vi "Update Method Result.vi"(8 "error in (no error)":errorcluster, 10 "Test Method Result":T1, 11 "Test Tree In":refnum<class "Test Result Tree V2.lvclass">) -> (0 "error out":errorcluster, 3 "Test Tree Out":refnum<class "Test Result Tree V2.lvclass">)   [LabVIEW 2020, in "Test Result Tree V2.lvclass"]
uses:
  Test Result Tree/Test Result Tree V2.lvclass
  C:/Git/astemes-lunit/source/Framework/Helper Classes/Test Tree/Test Tree.lvclass
  Framework/Result Types/Method Result/Method Result.ctl
  Result/Status.ctl
  Framework/Result Types/Assertion Result/Assertion Result.ctl
  Framework/Result Types/Assertion Result/Public/TypeDefs/Assertion Type.ctl
  Framework/Helper Classes/Test Tree/Test Tree.lvclass/Test Tree.ctl
  Test Result Tree/Test Result Tree V2.lvclass/Test Result Tree V2.ctl
  Framework/Result Types/Method Result/Method Result.lvlib
  Framework/Helper Classes/Test Tree/Test Tree.lvclass
  C:/Git/astemes-lunit/source/Rewrite Project/Test Result Tree/Test Result Tree/Test Result Tree V2.lvclass
  Framework/Result Types/Assertion Result/Assertion Result.lvlib
  Result/Result.lvlib
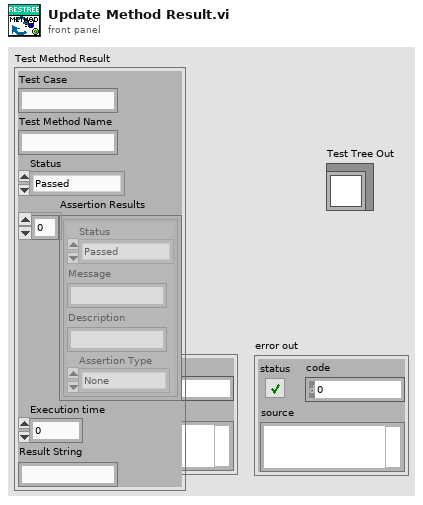
[diagram p1: front panel]
types:
  T1 = typedef "Method Result.lvlib/Method Result.ctl" = cluster{"Test Case":string, "Test Method Name":string, "Status":T2, "Assertion Results":T3[], "Execution time":dbl, "Result String":string}
  T2 = typedef "Result.lvlib/Status.ctl" = enum16{"Passed", "Failed", "Error", "Skipped", "Setup Error", "Broken", "Teardown Error"}
  T3 = typedef "Assertion Result.lvlib/Assertion Result.ctl" = cluster{"Status":T2, "Message":string, "Description":string, "Assertion Type":T4}
  T4 = typedef "Result.lvlib/Assertion Type.ctl" = enum16{"None", "Pass", "Fail", "Skip", "Pass if Equal", "Fail if Equal", "Pass if Error", "Fail if Error", "Pass if", "Fail if"}
  T5 = typedef "Assertion Result.lvlib/Status.ctl" = enum16{"Pass", "Fail", "Error", "Skipped", "Setup Error", "Broken", "Teardown Error"}
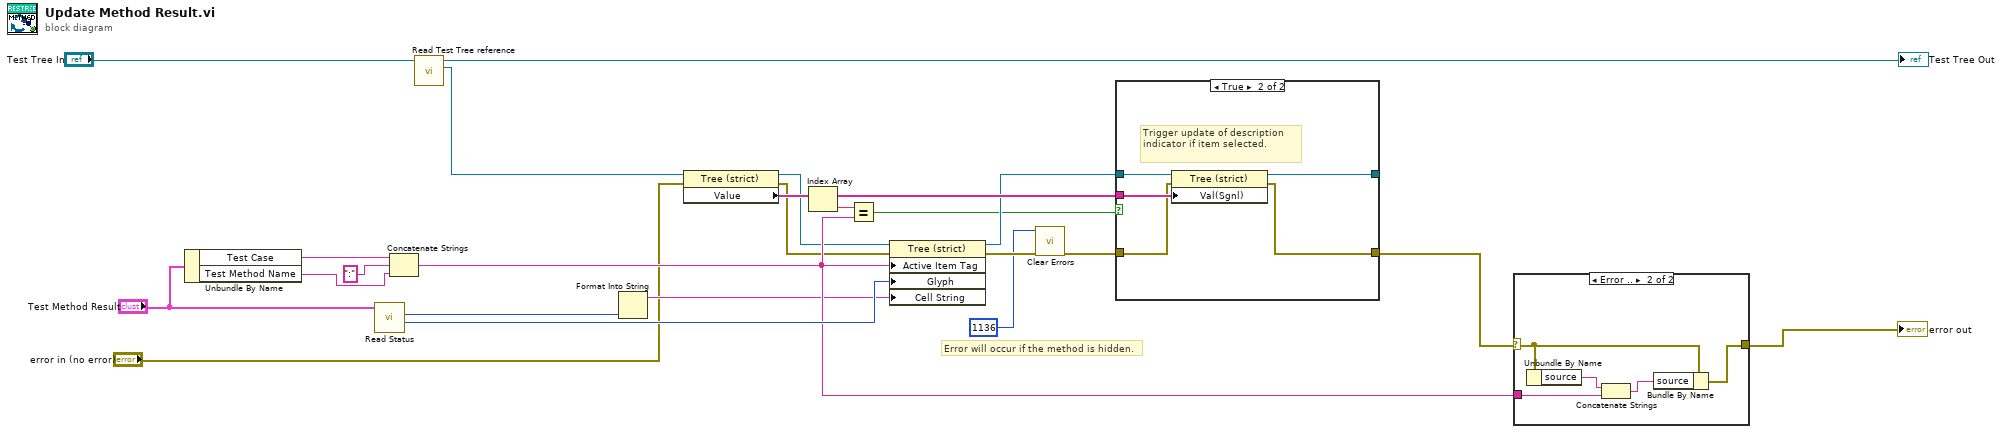
[diagram p0: block diagram]
diagram:
  # "Error will occur if the method is hidden."
  n1 = Unbundle By Name("Test Method Result") -> ("Test Case"=w1:string, "Test Method Name"=w2:string)
  n2 = call "Read Status.vi"("Method Result In"="Test Method Result") -> ("Glyph Index"=w21:i32, "Status"=w22:T5)  [unwired: 8 in, 1 out]
  n3 = Concatenate Strings(w1, ":" ("string"), w2) -> (w19:string)
  n4 = call "Read Test Tree reference.vi"("Test Tree in"="Test Tree In") -> ("Test Tree reference"=w5:refnum<vi>, "Test Tree out"=→"Test Tree Out":refnum<class "Test Result Tree V2.lvclass">)  [unwired: 8 in, 1 out]
  n5 = Format Into String(w22) -> (resulting string=w18:string)  [unwired: 3 in, 1 out]
  n6 = property on="Property Node" class="Tree (strict)"(reference=w5, error in="error in (no error)") -> (reference out=w11:refnum<vi>, error out=w12:errorcluster, "Value"=w16:string[])
  n7 = Index Array(array=w16) -> (element=w17:string)  [unwired: 1 in]
  n8 = Equal?(x=w17, y=w19) -> (x = y?=w10:bool)
  n9 = property class="Tree (strict)"(reference=w11, error in=w12, "Active Item Tag"=w19, "Glyph"=w21, "Cell String"=w18) -> (reference out=w15:refnum<vi>, error out=w14:errorcluster)
  n10 = call <vilib>:"Clear Errors.vi"("error in (no error)"=w14, "specific error code to clear (0: all)"=1136) -> ("error out"=w9:errorcluster)  [unwired: 4 in, 1 out]
  n11 = case shown="True" w10 {
    tunnel: w16 -> [_ w30]
    tunnel: w15 -> [w25 w29]
    tunnel: [w25 w28] -> _
    tunnel: w9 -> [w24 w27]
    tunnel: [w24 w26] -> w13
    frame False {
    }
    frame True {
      # "Trigger update of description indicator if item selected."
      n12 = property on="Property Node" class="Tree (strict)"(reference=w29, error in=w27, "Val(Sgnl)"=w30) -> (reference out=w28:refnum<vi>, error out=w26:errorcluster)
    }
  }
  n13 = case shown="Error .." w13 {
    selector: w13 -> [w31 w36]
    tunnel: [w31 w33] -> w20
    tunnel: w19 -> [_ w32]
    frame No Error {
    }
    frame Error {
      n14 = Unbundle By Name(w36) -> ("source"=w35:string)
      n15 = Concatenate Strings(w35, w32) -> (w34:string)
      n16 = Bundle By Name(cluster=w36, "source"=w34) -> (w33:errorcluster)
    }
  }
  "error out" <- w20
